vi "Find Folder Path.vi"(6 "File Name\nwith extension":string="Instruments", 8 "error in":errorcluster, 10 "Path\n(Empty at top level)":path, 11 "Config in":refnum<class "Config.lvclass">) -> (0 "error out":errorcluster, 2 "File Path Control":path, 3 "Config out":refnum<class "Config.lvclass">)   [LabVIEW 2023, in "Config.lvlib" / "Config.lvclass"]
uses:
  Config.lvclass
  <vilib>/Utility/sysdir.llb/System Directory Type.ctl
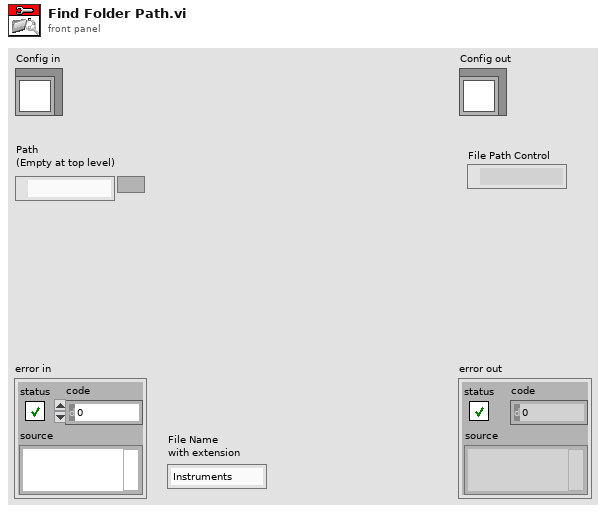
[diagram p1: front panel]
types:
  T1 = typedef "System Directory Type.ctl" = i32
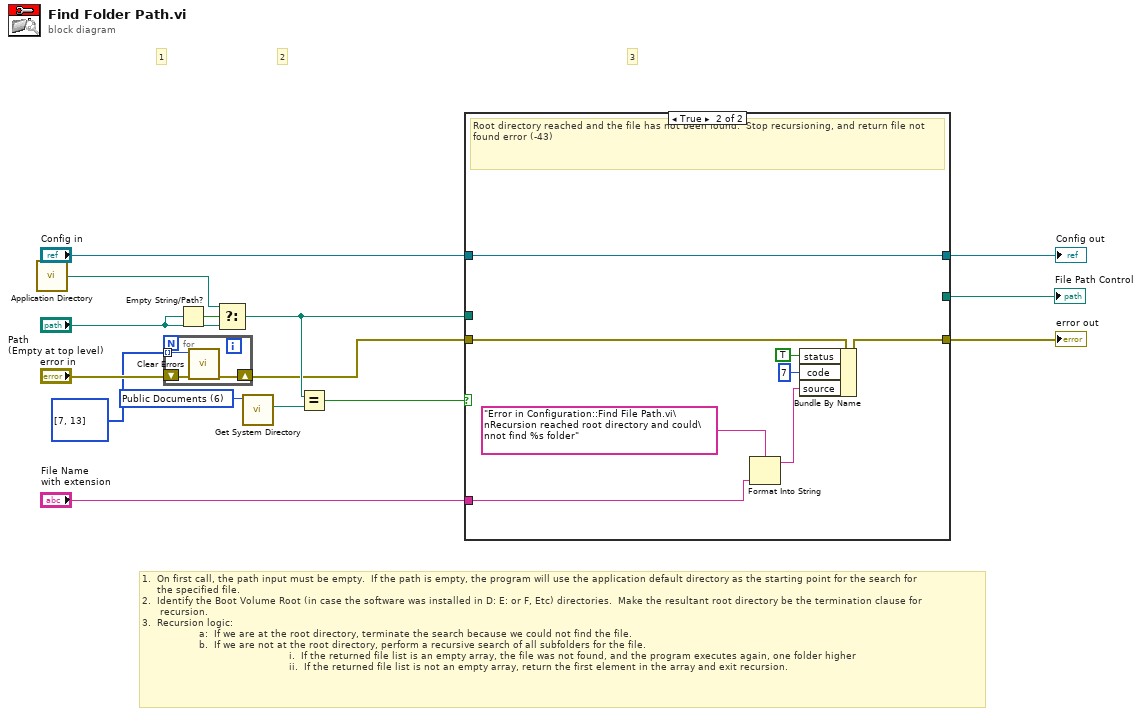
[diagram p0: block diagram]
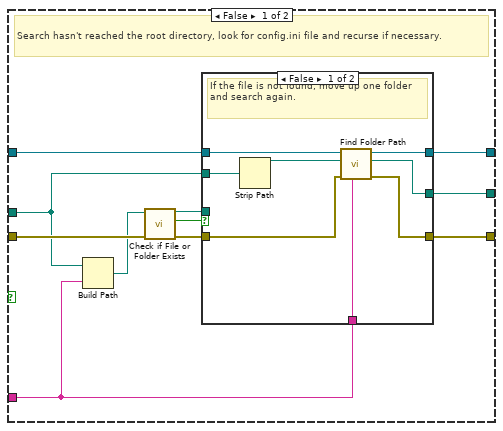
[diagram p2: hidden frame]
diagram:
  w9 = T1 6 items=["User Home"=0, "User Desktop"=1, "User Documents"=2, "User Application Data"=3, "User Preferences"=4, "User Temporary"=5, "Public Documents"=6, "Public Application Data"=7, "Public Preferences"=8, "Public Cache"=13, "System Core Libraries"=9, "System Installed Libraries"=10, "Application Files"=11, "Boot Volume Root"=12] ("system directory type")
  # "1.  On first call, the path input must be empty.  If the path is empty, the program will use the application default directory as the starting point for the search for\n     the specified file.\n2.  Identify the Boot Volume Root (in case the software was installed in D: E: or F, Etc) directories.  Make the resultant root directory be the termination clause for \n      recursion.\n3.  Recursion logic:  \n                   a:  If we are at the root directory, terminate the search because we could not find the file.\n                   b.  If we are not at the root directory, perform a recursive search of all subfolders for the file.  \n                                                 i.  If the returned file list is an empty array, the file was not found, and the program executes again, one folder higher\n                                                 ii.  If the returned file list is not an empty array, return the first element in the array and exit recursion."
  # "3"
  # "2"
  # "1"
  n1 = call <vilib>:"Application Directory.vi"() -> ("Application Directory"=w1:path)
  n2 = for {
    tunnel: i32[] [7, 13] -> [w16] mode=indexing
    shift-right: [w17] -> w3
    shift-left: "error in" -> [w18]
    n3 = call <vilib>:"Clear Errors.vi"("error in (no error)"=w18, "specific error code to clear (0: all)"=w16) -> ("error out"=w17:errorcluster)  [unwired: 4 in, 1 out]
  }
  n4 = Empty String/Path?(string/path="Path\n(Empty at top level)") -> (empty?=w15:bool)
  n5 = Select(t=w1, s=w15, f="Path\n(Empty at top level)") -> (s? t:f=w7:path)
  n6 = call <vilib>:"Get System Directory.vi"("system directory type"=w9) -> ("system directory"=w8:path)  [unwired: 10 in]
  n7 = Equal?(x=w7, y=w8) -> (x = y?=w6:bool)
  n8 = case shown="True" w6 {
    tunnel: "Config in" -> [w29 w48]
    tunnel: [w28 w48] -> w12
    tunnel: w3 -> [w24 w47]
    tunnel: [w27 w46] -> w10
    tunnel: w7 -> [w19 _]
    tunnel: "File Name\nwith extension" -> [w21 w42]
    tunnel: [w26 _] -> w4
    frame False {
      # "Search hasn't reached the root directory, look for config.ini file and recurse if necessary."
      n9 = Build Path(base path=w19, name or relative path=w21) -> (appended path=w20:path)
      n10 = call <vilib>:"Check if File or Folder Exists.vi"("error in (no error)"=w24, "path"=w20) -> ("error out"=w23:errorcluster, "file or folder exists?"=w22:bool, "dup path"=w25:path)  [unwired: 7 in]
      n11 = case shown="False" w22 {
        tunnel: w25 -> [_ w38]
        tunnel: w29 -> [w37 w39]
        tunnel: [w36 w39] -> w28
        tunnel: w23 -> [w35 w40]
        tunnel: [w34 w40] -> w27
        tunnel: w21 -> [w32 _]
        tunnel: [w31 w38] -> w26
        tunnel: w19 -> [w30 _]
        frame False {
          # "If the file is not found, move up one folder and search again."
          n12 = Strip Path(path=w30) -> (stripped path=w33:path)  [unwired: 1 out]
          n13 = call "Find Folder Path.vi"("File Name\nwith extension"=w32, "error in"=w35, "Path\n(Empty at top level)"=w33, "Config in"=w37) -> ("error out"=w34:errorcluster, "File Path Control"=w31:path, "Config out"=w36:refnum<class "Config.lvclass">)  [unwired: 5 in]
        }
        frame True {
          # "If the file is found, return the first instance of the file as the file path"
        }
      }
    }
    frame True {
      # "Root directory reached and the file has not been found.  Stop recursioning, and return file not found error (-43)"
      n14 = Format Into String(format string="Error in Configuration::Find File Path.vi\nRecursion reached root directory and could\nnot find %s folder" ("source"), w42) -> (resulting string=w41:string)  [unwired: 2 in, 1 out]
      n15 = Bundle By Name(cluster=w47, "status"=TRUE, "code"=7, "source"=w41) -> (w46:errorcluster)
    }
  }
  "error out" <- w10
  "Config out" <- w12
  "File Path Control" <- w4
